vi "FindChessboardCornersARGB.vi"(7 "Flags (Default - Adaptive Threshold, Normalize and Fast Check)":T3[](array[typedef])=[enum."CALIB_CB_ADAPTIVE_THRESH", enum."CALIB_CB_NORMALIZE_IMAGE", enum."CALIB_CB_FAST_CHECK"], 8 "error in (no error)":errorcluster, 10 "Chessboard Corners Info":T2, 11 "ARGB Image":refnum<data-value>) -> (0 "error out":errorcluster, 2 "Points":T1[](array[typedef]), 3 "ARGB Image (Duplicate)":refnum<data-value>)   [LabVIEW 2020, in "g_ar_toolkit.camera_calibration.lvlib"]
uses:
  g_ar_toolkit.camera_calibration.lvlib
  Find Chessboard Corners Flags.ctl
  Chessboard Corner Info.ctl
  g_ar_toolkit.common/Image Point (Float).ctl
  ca99938f-1423-42fb-b653-ffd1f73e2bb5.vi
  <vilib>/Utility/error.llb/Error Cluster From Error Code.vi
  g_ar_toolkit.common/g_ar_toolkit.common.lvlib
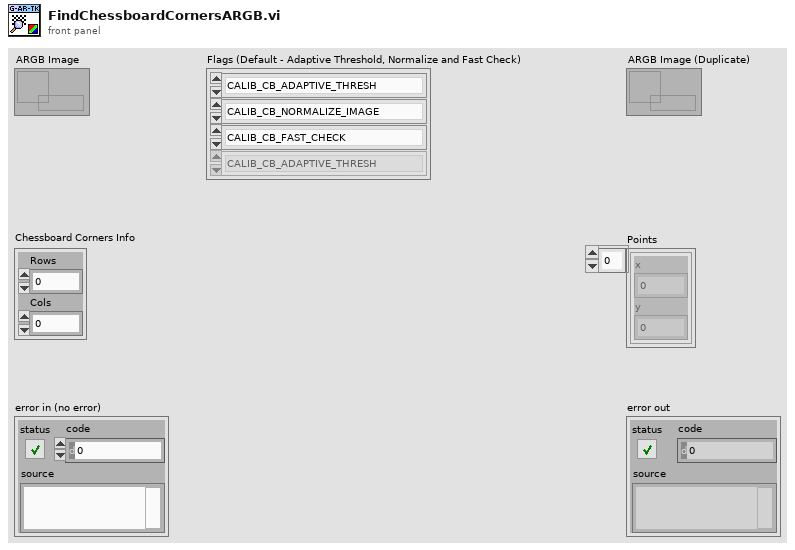
[diagram p1: front panel]
types:
  T1 = typedef "g_ar_toolkit.common.lvlib/Image Point (Float).ctl" = cluster{"x":dbl, "y":dbl}
  T2 = typedef "g_ar_toolkit.camera_calibration.lvlib/Chessboard Corner Info.ctl" = cluster{"Rows":u8, "Cols":u8}
  T3 = typedef "g_ar_toolkit.camera_calibration.lvlib/Find Chessboard Corners Flags.ctl" = enum16{"CALIB_CB_ADAPTIVE_THRESH", "CALIB_CB_NORMALIZE_IMAGE", "CALIB_CB_FILTER_QUADS", "CALIB_CB_FAST_CHECK"}
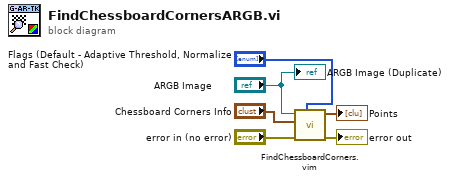
[diagram p0: block diagram]
diagram:
  n1 = call "FindChessboardCorners.vim"("Flags (Default - Adaptive Threshold, Normalize and Fast Check)"="Flags (Default - Adaptive Threshold, Normalize and Fast Check)", "error in (no error)"="error in (no error)", "Chessboard Corners Info"="Chessboard Corners Info", "Src"="ARGB Image") -> ("error out"=→"error out":errorcluster, "Points"=→"Points":cluster{"x":dbl, "y":dbl}[])  [unwired: 6 in]
  "ARGB Image (Duplicate)" <- "ARGB Image"
